vi "pollScan.vi"(8 "error in (no error)":errorcluster, 10 "Device":i32, 11 "Model in":refnum<class "Model.lvclass">) -> (0 "error out":errorcluster, 2 "Output Value":i32, 3 "Model out":refnum<class "Model.lvclass">)   [LabVIEW 2016, in "Model.lvclass"]
uses:
  Model.lvclass
  Model.lvclass/Model.ctl
  ss_sedspectrometer/SEDSpectrometer/SEDSpectrometer.lvclass
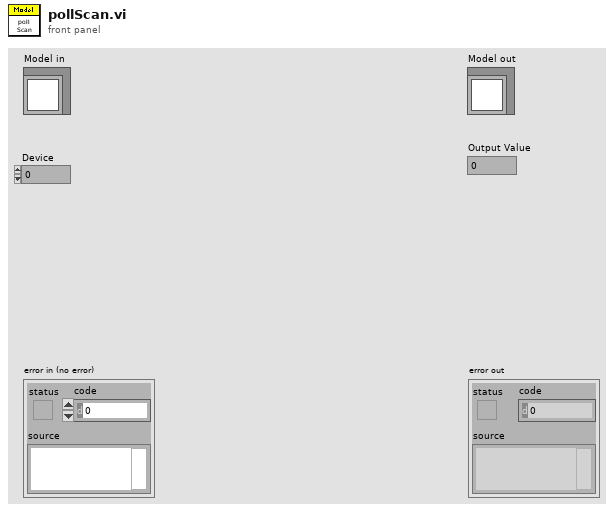
[diagram p1: front panel]
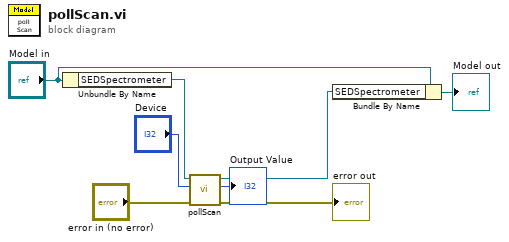
[diagram p0: block diagram]
diagram:
  n1 = Unbundle By Name("Model in") -> ("SEDSpectrometer"=w8:refnum<class "SEDSpectrometer.lvclass">)
  n2 = call "pollScan.vi"("error in (no error)"="error in (no error)", "Device"="Device", "SEDSpectrometer in"=w8) -> ("error out"=→"error out":errorcluster, "Output Value"=→"Output Value":i32, "SEDSpectrometer out"=w4:refnum<class "SEDSpectrometer.lvclass">)  [unwired: 6 in]
  n3 = Bundle By Name(cluster="Model in", "SEDSpectrometer"=w4) -> (→"Model out":refnum<class "Model.lvclass">)
